vi "erasechip.vi"   [LabVIEW 2011]
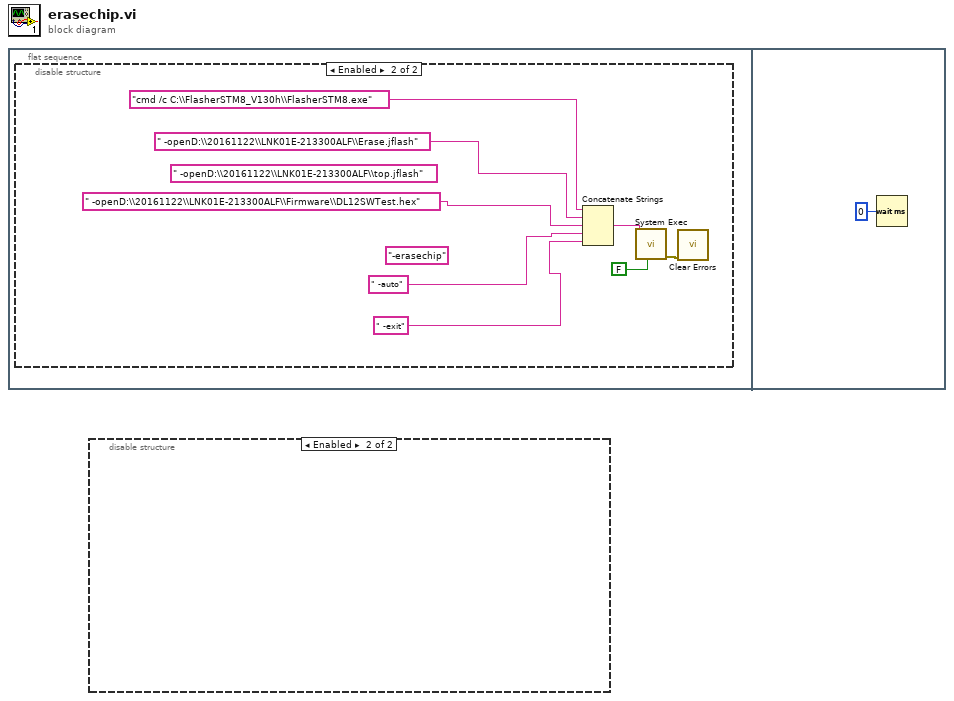
[diagram p0: block diagram]
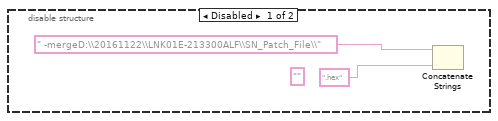
[diagram p2: hidden frame]
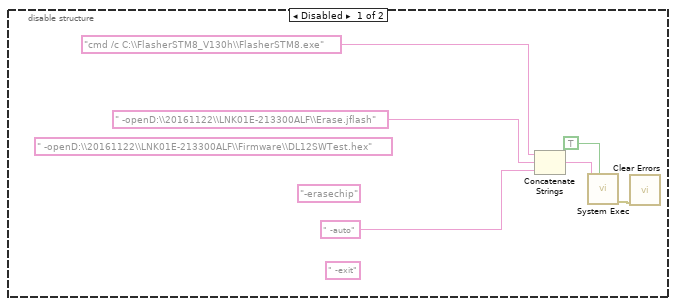
[diagram p3: hidden frame]
diagram:
  n1 = flat-sequence {
    frame #0 {
      n2 = disable-structure shown="Enabled" {
        frame Disabled {
          (unwired) "-erasechip" ("command line")
          (unwired) " -exit" ("command line")
          (unwired) " -openD:\\20161122\\LNK01E-213300ALF\\Firmware\\DL12SWTest.hex" ("command line")
          n3 = Concatenate Strings("cmd /c C:\\FlasherSTM8_V130h\\FlasherSTM8.exe" ("command line"), " -openD:\\20161122\\LNK01E-213300ALF\\Erase.jflash" ("command line"), " -auto" ("command line")) -> (w5:string)
          n4 = call <vilib>:"System Exec.vi"("wait until completion? (T)"=TRUE, "command line"=w5) -> ("error out"=w6:errorcluster)  [unwired: 6 in, 3 out]
          n5 = call <vilib>:"Clear Errors.vi"("error in (no error)"=w6) -> ()  [unwired: 5 in, 2 out]
        }
        frame Enabled {
          (unwired) "-erasechip" ("command line")
          (unwired) " -openD:\\20161122\\LNK01E-213300ALF\\top.jflash" ("command line")
          n6 = Concatenate Strings("cmd /c C:\\FlasherSTM8_V130h\\FlasherSTM8.exe" ("command line"), " -openD:\\20161122\\LNK01E-213300ALF\\Erase.jflash" ("command line"), " -openD:\\20161122\\LNK01E-213300ALF\\Firmware\\DL12SWTest.hex" ("command line"), " -auto" ("command line"), " -exit" ("command line")) -> (w12:string)
          n7 = call <vilib>:"System Exec.vi"("run minimized? (F)"=FALSE, "command line"=w12) -> ("error out"=w13:errorcluster)  [unwired: 6 in, 3 out]
          n8 = call <vilib>:"Clear Errors.vi"("error in (no error)"=w13) -> ()  [unwired: 5 in, 2 out]
        }
      }
    }
    frame #1 {
      n9 = Wait (ms)(milliseconds to wait=u32 0) -> ()  [unwired: 1 out]
    }
  }
  n10 = disable-structure shown="Enabled" {
    frame Disabled {
      (unwired) "" ("string")
      n11 = Concatenate Strings(" -mergeD:\\20161122\\LNK01E-213300ALF\\SN_Patch_File\\" ("command line"), ".hex" ("command line")) -> ()  [unwired: 1 in, 1 out]
    }
    frame Enabled {
    }
  }
